vi "tempeture conversions.vi"() -> ()   [LabVIEW 2014]
panel:
  out "output tempeture":dbl
  in  "input tempeture":dbl
  in  "Enum":enum16{"F to C", "C to F", "C to K", "F to K"}(ring)
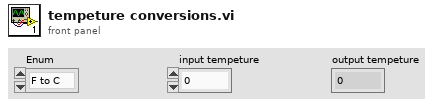
[diagram p1: front panel]
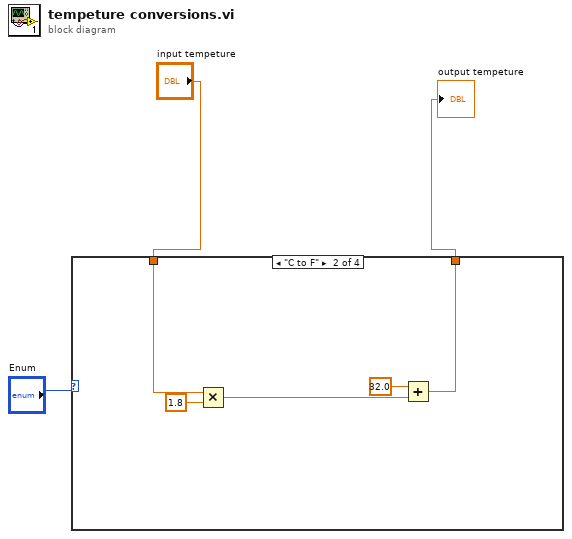
[diagram p0: block diagram]
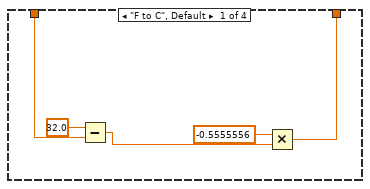
[diagram p2: hidden frame]
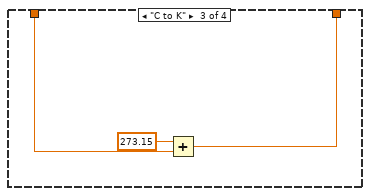
[diagram p3: hidden frame]
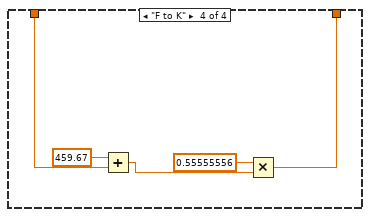
[diagram p4: hidden frame]
diagram:
  n1 = case shown="\"C to F\"" "Enum" {
    tunnel: "input tempeture" -> [w8 w11 w16 w21]
    tunnel: [w6 w12 w15 w19] -> w1
    frame "F to C", Default {
      n2 = Subtract(x=32.0, y=w8) -> (x-y=w7:dbl)
      n3 = Multiply(x=-0.5555556, y=w7) -> (x*y=w6:dbl)
    }
    frame "C to F" {
      n4 = Multiply(x=w11, y=1.8) -> (x*y=w13:dbl)
      n5 = Add(x=32.0, y=w13) -> (x+y=w12:dbl)
    }
    frame "C to K" {
      n6 = Add(x=273.15, y=w16) -> (x+y=w15:dbl)
    }
    frame "F to K" {
      n7 = Add(x=459.67, y=w21) -> (x+y=w20:dbl)
      n8 = Multiply(x=0.55555556, y=w20) -> (x*y=w19:dbl)
    }
  }
  "output tempeture" <- w1
